vi "HexTString.vi"(1 "input Hex":string) -> (0 "output string":string)   [LabVIEW 2010]
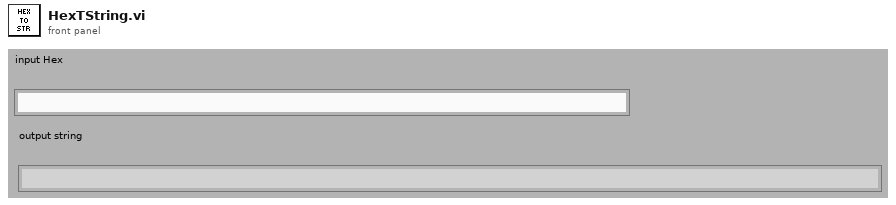
[diagram p1: front panel]
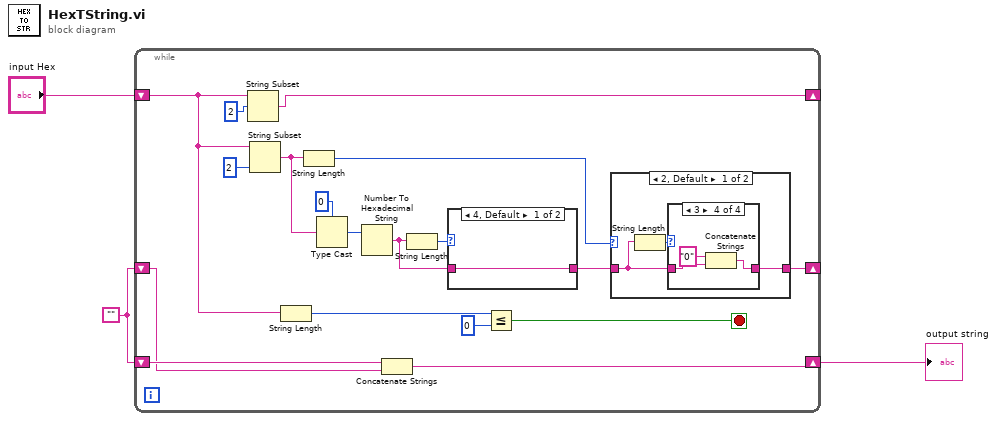
[diagram p0: block diagram]
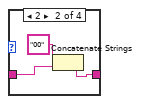
[diagram p3: hidden frame]
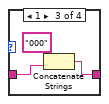
[diagram p4: hidden frame]
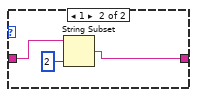
[diagram p5: hidden frame]
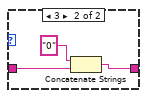
[diagram p6: hidden frame]
diagram:
  w3 = ""
  n1 = while {
    shift-right: [w19] -> _
    shift-left: "input Hex" -> [w9]
    shift-right: [w11] -> _
    shift-left: w3 -> [w4]
    shift-right: [w10] -> w1
    shift-left: w3 -> [w5]
    stop <- w6 stop-if-true
    n2 = String Subset(string=w9, offset (0)=2 ("长度（剩余）")) -> (substring=w19:string)  [unwired: 1 in]
    n3 = String Subset(string=w9, length (rest)=2 ("长度（剩余）")) -> (substring=w16:string)  [unwired: 1 in]
    n4 = String Length(string=w9) -> (length=w8:i32)
    n5 = String Length(string=w16) -> (length=w13:i32)
    n6 = Type Cast(type=u16 0, x=w16) -> (*(type *) &x=w17:u16)
    n7 = Number To Hexadecimal String(2:w17) -> (0:w14:string)  [unwired: 1 in]
    n8 = Concatenate Strings(w5, w4) -> (w10:string)
    n9 = String Length(string=w14) -> (length=w15:i32)
    n10 = case shown="4, Default" w15 {
      tunnel: w14 -> [w38 w41]
      tunnel: [w38 w39] -> w12
      frame 4, Default {
      }
      frame 3 {
        n11 = Concatenate Strings("0" ("字符串"), w41) -> (w39:string)
      }
    }
    n12 = Less Or Equal?(x=w8, y=0) -> (x <= y?=w6:bool)
    n13 = case shown="2, Default" w13 {
      tunnel: w12 -> [w23 w37]
      tunnel: [w22 w35] -> w11
      frame 2, Default {
        n14 = String Length(string=w23) -> (length=w24:i32)
        n15 = case shown="3" w24 {
          tunnel: [w25 w28 w29 w33] -> w22
          tunnel: w23 -> [w25 w27 w31 w34]
          frame 4, Default {
          }
          frame 2 {
            n16 = Concatenate Strings("00" ("字符串"), w27) -> (w28:string)
          }
          frame 1 {
            n17 = Concatenate Strings("000" ("字符串"), w31) -> (w29:string)
          }
          frame 3 {
            n18 = Concatenate Strings("0" ("字符串"), w34) -> (w33:string)
          }
        }
      }
      frame 1 {
        n19 = String Subset(string=w37, length (rest)=2 ("长度（剩余）")) -> (substring=w35:string)  [unwired: 1 in]
      }
    }
  }
  "output string" <- w1
